vi "tearDown.vi"(8 "error in (no error)":errorcluster, 11 "reference in":refnum<class "DFA Tester.lvclass">) -> (0 "error out":errorcluster, 3 "reference out":refnum<class "DFA Tester.lvclass">)   [LabVIEW 2016, in "Assert API Components.lvlib" / "Log Assert Core.lvlib" / "DFA Tester.lvclass"]
doc: "tearDown runs after the test method has completed. Use this method to clean up any operations or references that were opened by setUp or the test method. Unit tests should be independent of other unit tests so this VI should ensure that the next test can run in a 'clean' test environment."
uses:
  DFA Tester.lvclass
  DFA Tester.lvclass/DFA Tester.ctl
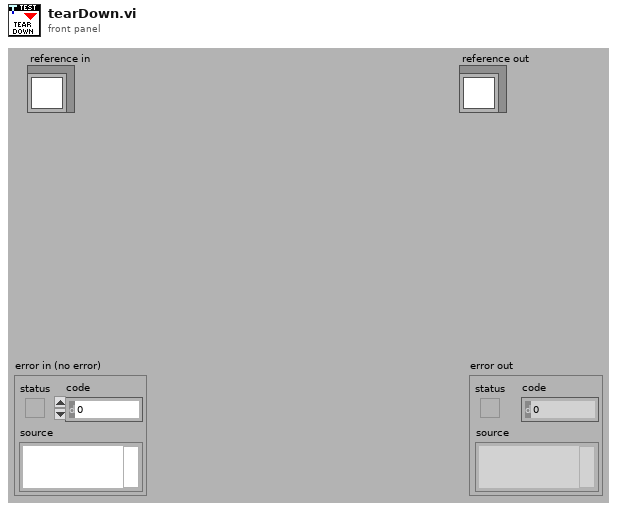
[diagram p1: front panel]
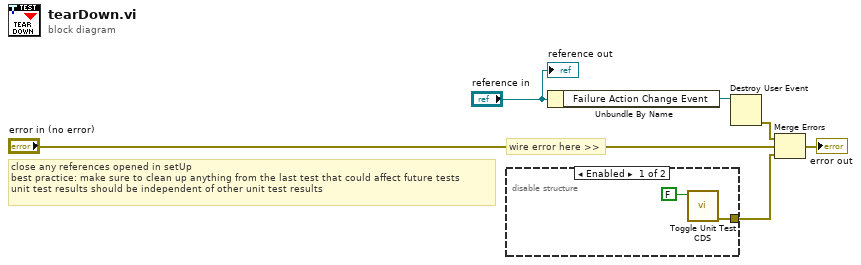
[diagram p0: block diagram]
diagram:
  # "wire error here >>"
  # "close any references opened in setUp\nbest practice: make sure to clean up anything from the last test that could affect future tests\nunit test results should be independent of other unit test results"
  n1 = disable-structure shown="Enabled" {
    disable-tunnel: [w7 _] -> w1
    frame Enabled {
      n2 = call "Toggle Unit Test CDS.vi"("Requested State"=FALSE) -> ("error out"=w7:errorcluster)  [unwired: 10 in]
    }
    frame Disabled {
    }
  }
  n3 = Unbundle By Name("reference in") -> ("Failure Action Change Event"=w3:refnum<user-event>)
  n4 = Destroy User Event(user event=w3) -> (error out=w2:errorcluster)  [unwired: 1 in]
  n5 = Merge Errors(w2, "error in (no error)", w1) -> (→"error out":errorcluster)
  "reference out" <- "reference in"
